vi "PH_HamamatsuCamera.get Basic Cam Information.vi"(0 "i ref in":refnum<vi>, 1 "Cam Handle in":i32, 4 "Cam Error in":errorcluster, 5 "error in (no error)":errorcluster) -> (14 "i ref out":refnum<vi>, 15 "Cam Handle out":i32, 18 "Cam Error out":errorcluster, 19 "error out":errorcluster)   [LabVIEW 2014, in "PH_HamamatsuCamera.lvlib"]
doc: "This VI gets basic camara information which has to got only once and saves it to own attributes and shows it in different GUI elements."
uses:
  PH_HamamatsuCamera.lvlib
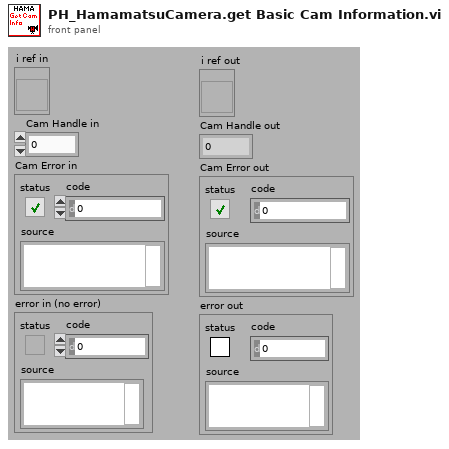
[diagram p1: front panel]
types:
  T1 = cluster{"Mode":u32, "Polarity":u32, "Times":u32, "Delay":dbl}
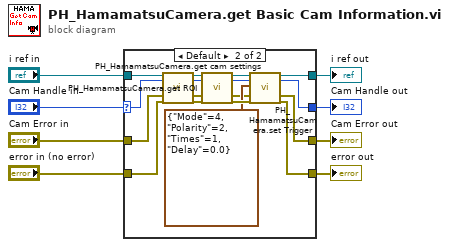
[diagram p0: block diagram]
diagram:
  n1 = case shown="Default" "Cam Handle in" {
    selector: "Cam Handle in" -> [w11 w13]
    tunnel: [w12 w29] -> w8
    tunnel: [w9 w28] -> w7
    tunnel: "i ref in" -> [w12 w27]
    tunnel: "error in (no error)" -> [w9 w26]
    tunnel: [w10 w16] -> w4
    tunnel: [w11 w15] -> w3
    tunnel: "Cam Error in" -> [w10 w14]
    frame -1 {
    }
    frame Default {
      n2 = call "PH_HamamatsuCamera.get cam settings.vi"("i ref in"=w27, "Cam Handle in"=w13, "Cam Error in"=w14, "error in (no error)"=w26) -> ("i ref out"=w22:refnum<vi>, "Handle out"=w19:i32, "Cam Error out"=w20:errorcluster, "error out"=w21:errorcluster)  [unwired: 12 in]
      n3 = call "PH_HamamatsuCamera.get ROI.vi"("i ref in"=w22, "Cam Handle in"=w19, "Cam Error in"=w20, "error in (no error)"=w21) -> ("i ref out"=w25:refnum<vi>, "Handle out"=w17:i32, "Cam Error out"=w18:errorcluster, "error out"=w24:errorcluster)  [unwired: 12 in]
      n4 = call "PH_HamamatsuCamera.set Trigger.vi"("i ref in"=w25, "Cam Handle in"=w17, "Trigger Parameters"=T1 {"Mode"=4, "Polarity"=2, "Times"=1, "Delay"=0.0}, "Cam Error in"=w18, "error in (no error)"=w24) -> ("i ref out"=w29:refnum<vi>, "Cam Handle out"=w15:i32, "Cam Error out"=w16:errorcluster, "error out"=w28:errorcluster)  [unwired: 11 in]
    }
  }
  "i ref out" <- w8
  "error out" <- w7
  "Cam Error out" <- w4
  "Cam Handle out" <- w3
